vi "test_stackHorizontally.vi"(11 "Test Case In":refnum<class "StackTests.lvclass">) -> (0 "error out":errorcluster, 3 "Test Case Out":refnum<class "StackTests.lvclass">)   [LabVIEW 2023, in "StackTests.lvclass"]
uses:
  StackTests.lvclass
  source/Ctrls/alignment.ctl
  <vilib>/Astemes/LUnit/Test Case.lvclass/Test Case.ctl
  <vilib>/Astemes/LUnit/Core/LUnit Test Case/Private/Append Fail Result.vi
  <vilib>/Astemes/LUnit/Core/LUnit Test Case/Private/Append Pass Result.vi
  <vilib>/Astemes/LUnit/Core/LUnit Test Case/Private/Run In UI.vi
  <vilib>/Utility/error.llb/Clear Errors.vi
  StackTests.lvclass/StackTests.ctl
  <vilib>/Astemes/LUnit/Test Case.lvclass
panel:
  in  "Numeric":dbl
  in  "btn":bool
  in  "firstItem":string
  in  "String":string
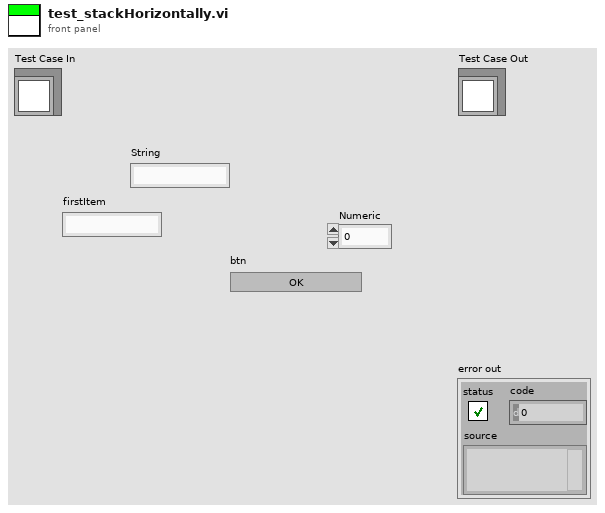
[diagram p1: front panel]
types:
  T1 = typedef "alignment.ctl" = enum16{"None", "AlignTop", "AlignBottom", "AlignHorizontalCenters", "AlignLeft", "AlignRight", "AlignVerticalCenters"}
  T2 = typedef "LVPositionTypeDef.ctl" = cluster{"Left":i32, "Top":i32}
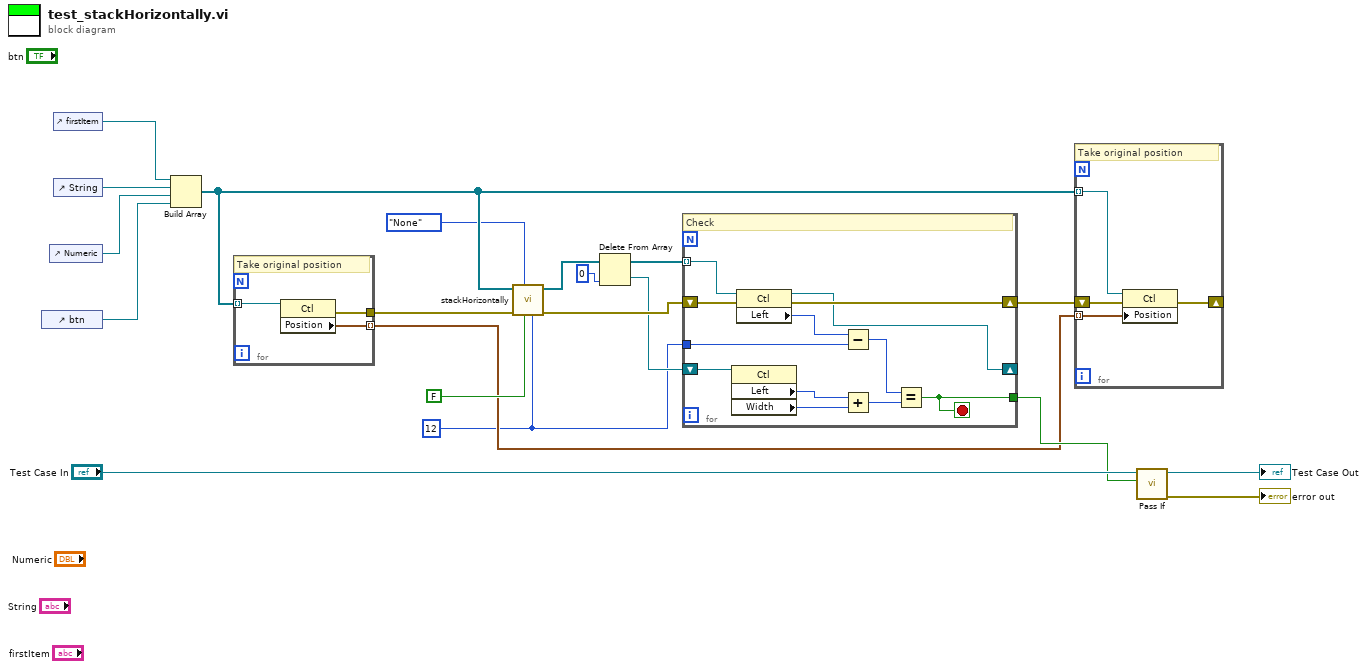
[diagram p0: block diagram]
diagram:
  w4 = u16 12 ("spacing")
  n1 = control-ref of="btn"() -> (w2:refnum<vi>)
  n2 = control-ref of="Numeric"() -> (w3:refnum<vi>)
  n3 = control-ref of="firstItem"() -> (w17:refnum<vi>)
  n4 = control-ref of="String"() -> (w16:refnum<vi>)
  n5 = Build Array(w17, w16, w3, w2) -> (w7:refnum<vi>[])
  n6 = for {
    tunnel: w7 -> [w23] mode=indexing
    tunnel: [w22] -> w5 mode=indexing
    tunnel: [w21] -> w15
    # "Take original position"
    n7 = property class="Ctl"(reference=w23) -> (error out=w21:errorcluster, "Position"=w22:T2)  [unwired: 1 in, 1 out]
  }
  n8 = call "stackHorizontally.vi"("spacing"=w4, "useControlBodyOnly"=FALSE, "verticalAlignment"=alignment."None", "error in (no error)"=w15, "refs"=w7) -> ("error out"=w13:errorcluster, "refs(dup)"=w10:refnum<vi>[])  [unwired: 5 in]
  n9 = Delete From Array(array=w10, index=0) -> (deleted portion=w11:refnum<vi>, array with subset deleted=w9:refnum<vi>[])  [unwired: 1 in]
  n10 = for {
    tunnel: w9 -> [w35] mode=indexing
    shift-right: [w33] -> w8
    shift-left: w13 -> [w34]
    shift-right: [w31] -> _
    shift-left: w11 -> [w32]
    tunnel: [w27] -> w6
    tunnel: w4 -> [w24]
    stop <- w27 stop-if-true
    # "Check"
    n11 = property class="Ctl"(reference=w32) -> ("Left"=w30:i32, "Width"=w29:u32)  [unwired: 1 in, 2 out]
    n12 = property class="Ctl"(reference=w35, error in=w34) -> (reference out=w31:refnum<vi>, error out=w33:errorcluster, "Left"=w26:i32)
    n13 = Subtract(x=w26, y=w24) -> (x-y=w25:i32)
    n14 = Add(x=w30, y=w29) -> (x+y=w28:u32)
    n15 = Equal?(x=w25, y=w28) -> (x = y?=w27:bool)
  }
  n16 = for {
    tunnel: w7 -> [w39] mode=indexing
    tunnel: w5 -> [w38] mode=indexing
    shift-right: [w37] -> _
    shift-left: w8 -> [w36]
    # "Take original position"
    n17 = property class="Ctl"(reference=w39, error in=w36, "Position"=w38) -> (error out=w37:errorcluster)  [unwired: 1 out]
  }
  n18 = call <vilib>:"Pass If.vi"("Pass?"=w6, "LUnit Test Case In"="Test Case In") -> ("error out"=→"error out":errorcluster, "LUnit Test Case Out"=→"Test Case Out":refnum<class "StackTests.lvclass">)  [unwired: 8 in]
